vi "利用数列计算PI值.vi"() -> (3 "PI":dbl format="%#_10g")   [LabVIEW 2012]
doc: "功能：\n\n利用数列求PI值。\n\n数列：\n\nPI/4=1/1-1/3+1/5-1/7.....\n\nCSXCS_366创建"
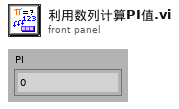
[diagram p1: front panel]
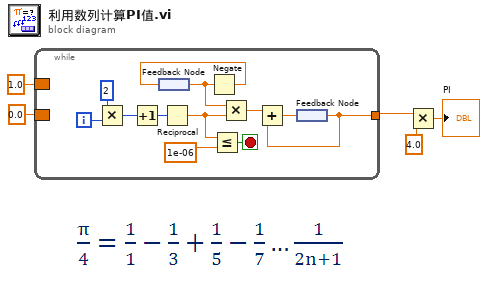
[diagram p0: block diagram]
diagram:
  n1 = while {
    tunnel: [w6] -> w3
    border: 1.0 -> [_]
    border: 0.0 -> [_]
    i -> [w17]
    stop <- w13 stop-if-true
    n2 = Multiply(x=2, y=w17) -> (x*y=w15:i32)
    n3 = Increment(x=w15) -> (x+1=w14:i32)
    n4 = feedback #1() -> (w8:dbl)
    n5 = Reciprocal(x=w14) -> (1/x=w11:dbl)
    n6 = Negate(x=w8) -> (-x=w9:dbl)
    n7 = feedback-in #1(w9) -> ()
    n8 = Less Or Equal?(x=w11, y=1e-06) -> (x <= y?=w13:bool)
    n9 = Multiply(x=w8, y=w11) -> (x*y=w12:dbl)
    n10 = feedback #2() -> (w6:dbl)
    n11 = Add(x=w12, y=w6) -> (x+y=w7:dbl)
    n12 = feedback-in #2(w7) -> ()
  }
  n13 = Multiply(x=w3, y=4.0) -> (x*y=→"PI":dbl)
